vi "Get Display Colours.vi"(8 "error in (no error)":errorcluster, 11 "Standard Display Configuration in":refnum<class "Standard Display Configuration.lvclass">) -> (0 "error out":errorcluster, 3 "Standard Display Configuration out":refnum<class "Standard Display Configuration.lvclass">)   [LabVIEW 2016, in "Assert API Components.lvlib" / "Assert Display.lvlib" / "Main Display.lvlib" / "Standard Display Configuration.lvclass"]
uses:
  Standard Display Configuration.lvclass
  D:/Work/Projects/actor_assert_api/Main Display/Display Configurations/Base Display Configuration.lvclass
  Main Display/Display Colours.ctl
  Base Display Configuration.lvclass/Base Display Configuration.ctl
  <vilib>/Utility/config.llb/Read Key (Boolean).vi
  <vilib>/Utility/config.llb/Read Key (U32).vi
  Assert API Components/Assert API Components.lvlib
  <vilib>/Utility/config.llb/NI_LVConfig.lvlib
  Base Display Configuration.lvclass
  Main Display.lvlib
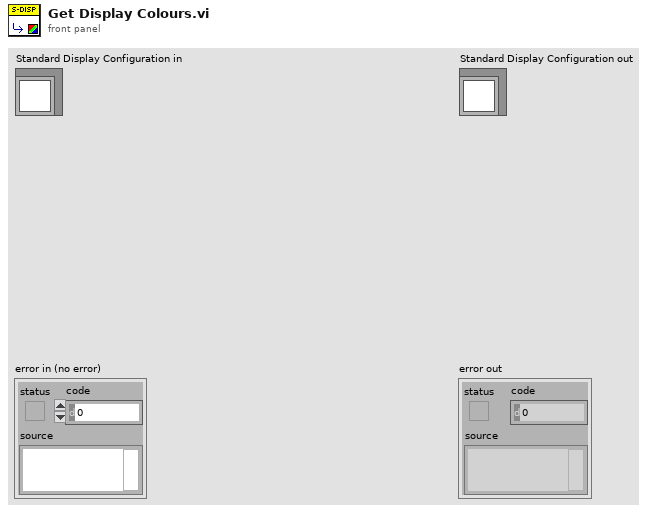
[diagram p1: front panel]
types:
  T1 = typedef "Assert API Components.lvlib/Assert Display.lvlib/Main Display.lvlib/Display Colours.ctl" = cluster{"Enable Colours":bool, "Passed Colour":u32, "Failed Colour":u32}
  T2 = typedef "NI_LVConfig.lvlib/Config Data RefNum.ctl" = refnum<k1>
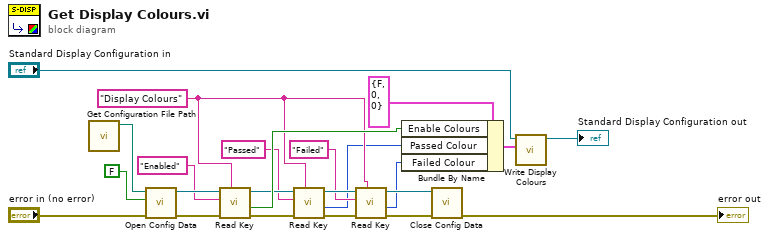
[diagram p0: block diagram]
diagram:
  w9 = "Display Colours" ("section")
  n1 = call "Get Configuration File Path.vi"() -> ("Configuration File Path"=w22:path)  [unwired: 11 in]
  n2 = call <vilib>:"Open Config Data.vi"("error in (no error)"="error in (no error)", "create file if necessary (T)"=FALSE, "configuration file path"=w22) -> ("error out"=w20:errorcluster, "refnum"=w21:T2)  [unwired: 6 in, 1 out]
  n3 = call-poly <vilib>:"Read Key.vi"("section"=w9, "error in (no error)"=w20, "key"="Enabled", "refnum"=w21) -> ("error out"=w19:errorcluster, "value"=w17:bool, "refnum out"=w15:T2)  [unwired: 4 in, 1 out]
  n4 = call-poly <vilib>:"Read Key.vi"("section"=w9, "error in (no error)"=w19, "key"="Passed", "refnum"=w15) -> ("error out"=w16:errorcluster, "value"=w6:u32, "refnum out"=w13:T2)  [unwired: 4 in, 1 out]
  n5 = call-poly <vilib>:"Read Key.vi"("section"=w9, "error in (no error)"=w16, "key"="Failed", "refnum"=w13) -> ("error out"=w14:errorcluster, "value"=w5:u32, "refnum out"=w12:T2)  [unwired: 4 in, 1 out]
  n6 = Bundle By Name(cluster=T1 {"Enable Colours"=FALSE, "Passed Colour"=0, "Failed Colour"=0} ("Display Colours"), "Enable Colours"=w17, "Passed Colour"=w6, "Failed Colour"=w5) -> (w1:T1)
  n7 = call <vilib>:"Close Config Data.vi"("error in (no error)"=w14, "refnum"=w12) -> ("error out"=→"error out":errorcluster)  [unwired: 8 in, 1 out]
  n8 = call "Write Display Colours.vi"("Display Colours"=w1, "Base Display Configuration in"="Standard Display Configuration in") -> ("Base Display Configuration out"=→"Standard Display Configuration out":refnum<class "Standard Display Configuration.lvclass">)  [unwired: 9 in]
